vi "ReversedEngineering CountNoOfPathInPathArray.vi"(1 "Path":path, 2 "Path array":path[](array[path]), 5 "error in (no error)":errorcluster) -> (15 "noOfFounds":u32, 16 "anyFound":bool, 19 "error out":errorcluster)   [LabVIEW 2020]
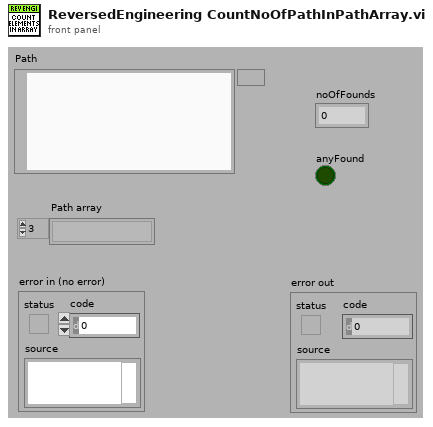
[diagram p1: front panel]
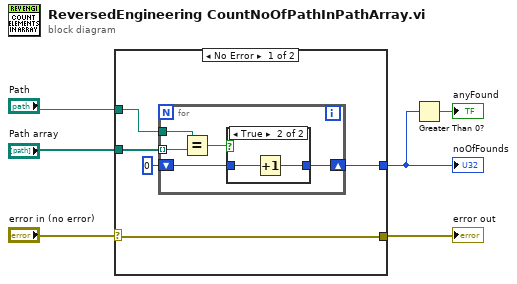
[diagram p0: block diagram]
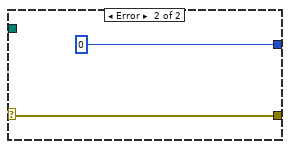
[diagram p3: hidden frame]
diagram:
  n1 = case shown="No Error" "error in (no error)" {
    selector: "error in (no error)" -> [w11 w21]
    tunnel: "Path" -> [w7 _]
    tunnel: [w11 w21] -> w5
    tunnel: "Path array" -> [w9 _]
    tunnel: [w8 u32 0] -> w2
    frame No Error {
      n2 = for {
        tunnel: w9 -> [w16] mode=indexing
        tunnel: w7 -> [w15]
        shift-right: [w12] -> w8
        shift-left: u32 0 -> [w13]
        n3 = Equal?(x=w15, y=w16) -> (x = y?=w14:bool)
        n4 = case shown="True" w14 {
          tunnel: w13 -> [w17 w19]
          tunnel: [w17 w18] -> w12
          frame False {
          }
          frame True {
            n5 = Increment(x=w19) -> (x+1=w18:u32)
          }
        }
      }
    }
    frame Error {
    }
  }
  "error out" <- w5
  "noOfFounds" <- w2
  n6 = Greater Than 0?(x=w2) -> (x > 0?=→"anyFound":bool)
